vi "trackTimer.vi"(8 "error in (no error)":errorcluster, 10 "Wheel Stripe Counter":u32, 11 "Time Target (s)":dbl) -> (0 "error out":errorcluster, 2 "Time has Elapsed":bool, 3 "Elapsed Time (s)":dbl)   [LabVIEW 2017]
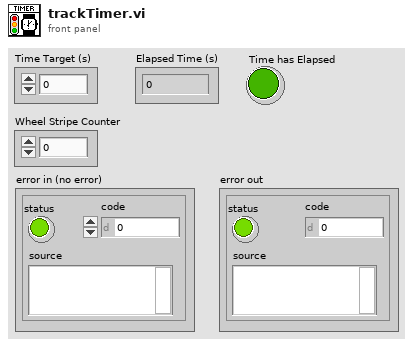
[diagram p1: front panel]
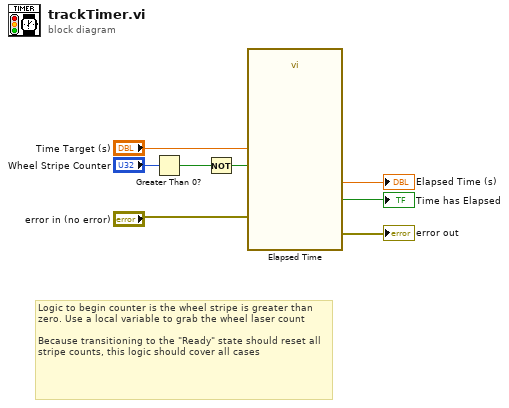
[diagram p0: block diagram]
diagram:
  # "Logic to begin counter is the wheel stripe is greater than zero. Use a local variable to grab the wheel laser count\n\nBecause transitioning to the \"Ready\" state should reset all stripe counts, this logic should cover all cases"
  n1 = Greater Than 0?(x="Wheel Stripe Counter") -> (x > 0?=w4:bool)
  n2 = Not(x=w4) -> (.not. x?=w3:bool)
  n3 = call "Elapsed Time"("Time Target (s)"="Time Target (s)", "Reset"=w3, "error in (no error)"="error in (no error)") -> ("Elapsed Time (s)"=→"Elapsed Time (s)":dbl, "Time has Elapsed"=→"Time has Elapsed":bool, "error out"=→"error out":errorcluster)  [unwired: 9 in, 5 out]
